vi "StartData.vi"(8 "error in (no error)":errorcluster, 11 "Class In":refnum<class "C37.118 PMU.lvclass">) -> (0 "error out":errorcluster, 3 "Class Out":refnum<class "C37.118 PMU.lvclass">)   [LabVIEW 2014, in "SensorPlugins.lvlib" / "C37.118 PMU.lvclass"]
uses:
  C37.118 PMU.lvclass
  Typedef/eCmdTypes.ctl
  C37.118 PMU.lvclass/C37.118 PMU.ctl
  <userlib>/NIST/Socket Class/Classes/Socket.Base/Socket.Base.lvclass/Socket.Base.ctl
  <userlib>/NIST/Socket Class/Classes/Socket.Base/Accessors/Read connected.vi
  Accessors/Read PMUConfigData.vi
  Accessors/Read CmdSocket.vi
  Accessors/Read PMUComms.vi
  Accessors/Read DataSocket.vi
  Accessors/Write CmdSocket.vi
  Accessors/Write DataSocket.vi
  <userlib>/NIST/Socket Class/Classes/Socket.Base/Socket.Base.lvclass
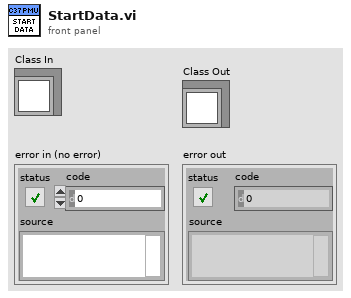
[diagram p1: front panel]
types:
  T1 = typedef "SensorPlugins.lvlib/C37.118 PMU.lvclass/eCmdTypes.ctl" = enum16{"Stop realtime data", "Start realtime data", "Send HDR file", "Send CFG-1 file", "Send CFG-2 file"}
  T2 = typedef "SensorPlugins.lvlib/C37.118 PMU.lvclass/PMUConfigData.ctl" = cluster{"TimeBase":u32, "NUM_PMU":u16, "Station Name":string, "IDCODE":u16, "PHRNMR":u16, "ANNMR":u16, "DIGNMR":u16, "FORMAT BITS":T3, "Valid Inputs":u16[], "DigitalStatusMask":u16[], "24bit_PHUNIT":i32[], "24bit_ANUNIT":u32[], "Analog Amplitude Setting":u32[], "Unit (Vor I)":u8[], "ChannelNames":string, "Fs":i16, "SOC ":u32, "FRACSEC":u32, "F0":sgl, "CFGCNT":u16}
  T3 = typedef "SensorPlugins.lvlib/C37.118 PMU.lvclass/FormatBits.ctl" = cluster{"Rect/Polar":bool, "Phasor Int/Float":bool, "Analog Int/Float":bool, "F/ROCOF Int/Float":bool}
  T4 = typedef "SensorPlugins.lvlib/C37.118 PMU.lvclass/PMUComms.ctl" = cluster{"PMU IP Address":string, "CMD Comms Type":T5, "Data Comms Type":T5, "CMD Port":u16, "Data Port":u16, "PMU ID":u16}
  T5 = typedef "SensorPlugins.lvlib/C37.118 PMU.lvclass/eCommsType.ctl" = enum16{"TCP", "UDP", "USB", "GPIB"}
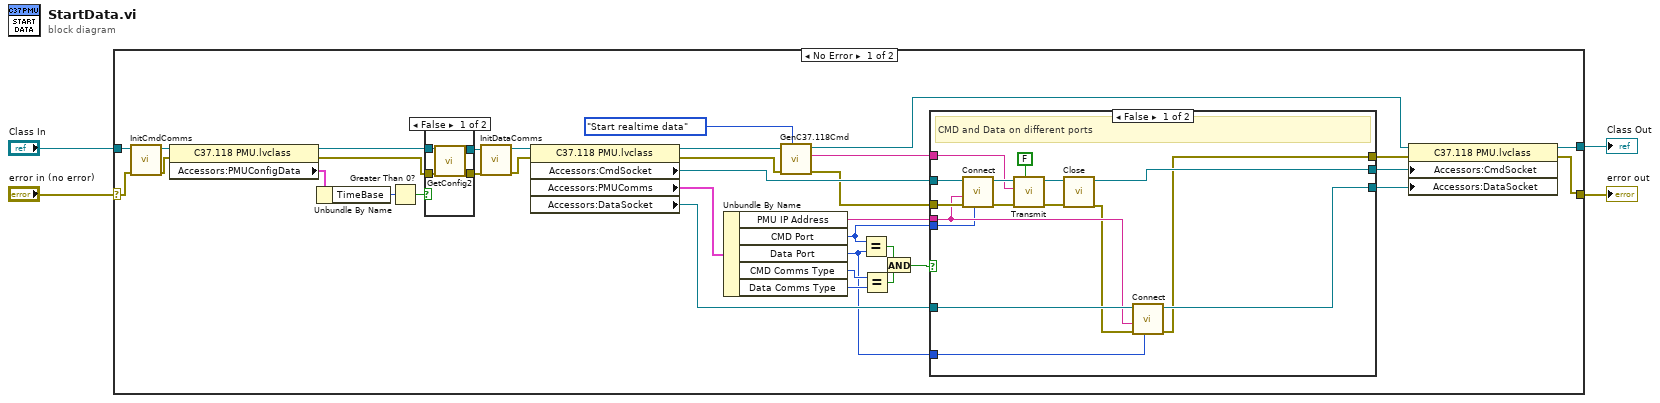
[diagram p0: block diagram]
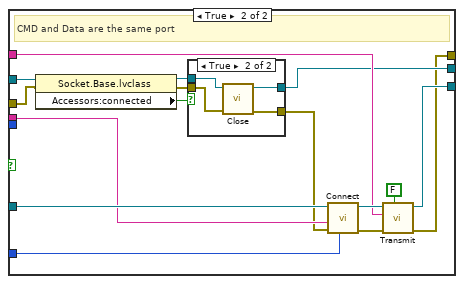
[diagram p3: hidden frame]
diagram:
  n1 = case shown="No Error" "error in (no error)" {
    selector: "error in (no error)" -> [w32 w84]
    tunnel: "Class In" -> [w33 w85]
    tunnel: [w28 w85] -> w2
    tunnel: [w23 w84] -> w1
    frame No Error {
      n2 = call "InitCmdComms.vi"("error in (no error)"=w32, "C37.118 PMU in"=w33) -> ("error out"=w7:errorcluster, "C37.118 PMU out"=w31:refnum<class "C37.118 PMU.lvclass">)  [unwired: 8 in]
      n3 = property class="C37.118 PMU.lvclass"(reference=w31, error in=w7) -> (reference out=w10:refnum<class "C37.118 PMU.lvclass">, error out=w6:errorcluster, "Accessors:PMUConfigData"=w12:T2)
      n4 = Unbundle By Name(w12) -> ("TimeBase"=w9:u32)
      n5 = Greater Than 0?(x=w9) -> (x > 0?=w8:bool)
      n6 = case shown="False" w8 {
        tunnel: [w43 w45] -> w11
        tunnel: w10 -> [w42 w45]
        tunnel: w6 -> [w41 w44]
        tunnel: [w40 w44] -> w5
        frame False {
          n7 = call "GetConfig2.vi"("error in (no error)"=w41, "C37.118 PMU in"=w42) -> ("error out"=w40:errorcluster, "C37.118 PMU out"=w43:refnum<class "C37.118 PMU.lvclass">)  [unwired: 8 in]
        }
        frame True {
        }
      }
      n8 = call "InitDataComms.vi"("error in (no error)"=w5, "C37.118 PMU in"=w11) -> ("error out"=w29:errorcluster, "C37.118 PMU out"=w30:refnum<class "C37.118 PMU.lvclass">)  [unwired: 8 in]
      n9 = property class="C37.118 PMU.lvclass"(reference=w30, error in=w29) -> (reference out=w38:refnum<class "C37.118 PMU.lvclass">, error out=w25:errorcluster, "Accessors:CmdSocket"=w37:refnum<class "Socket.Base.lvclass">, "Accessors:PMUComms"=w36:T4, "Accessors:DataSocket"=w26:refnum<class "Socket.Base.lvclass">)
      n10 = Unbundle By Name(w36) -> ("PMU IP Address"=w24:string, "CMD Port"=w15:u16, "Data Port"=w14:u16, "CMD Comms Type"=w20:T5, "Data Comms Type"=w19:T5)
      n11 = call "GenC37.118Cmd.vi"("Function"=eCmdTypes."Start realtime data", "error in (no error)"=w25, "PMUClass"=w38) -> ("error out"=w34:errorcluster, "Command"=w35:string, "PMUClass"=w13:refnum<class "C37.118 PMU.lvclass">)  [unwired: 6 in]
      n12 = Equal?(x=w15, y=w14) -> (x = y?=w18:bool)
      n13 = Equal?(x=w20, y=w19) -> (x = y?=w17:bool)
      n14 = And(x=w18, y=w17) -> (x .and. y?=w16:bool)
      n15 = case shown="False" w16 {
        tunnel: w37 -> [w61 w71]
        tunnel: w35 -> [w57 w72]
        tunnel: w34 -> [w56 w70]
        tunnel: [w53 w66] -> w27
        tunnel: w26 -> [w52 w77]
        tunnel: w24 -> [w51 w75]
        tunnel: [w50 w63] -> w22
        tunnel: [w48 w62] -> w21
        tunnel: w15 -> [w47 _]
        tunnel: w14 -> [w46 w76]
        frame False {
          # "CMD and Data on different ports"
          n16 = call-dynamic "Connect.vi"("remote_port"=w47, "error in (no error)"=w56, "remote_address"=w51, "Socket.Base in"=w61) -> ("error out"=w58:errorcluster, "Socket.Base out"=w59:refnum<class "Socket.Base.lvclass">)  [unwired: 6 in]
          n17 = call-dynamic "Transmit.vi"("packet? (f)"=FALSE, "error in (no error)"=w58, "data"=w57, "Socket.Base in"=w59) -> ("error out"=w55:errorcluster, "Socket.Base out"=w54:refnum<class "Socket.Base.lvclass">)  [unwired: 5 in, 1 out]
          n18 = call-dynamic "Close.vi"("error in (no error)"=w55, "Socket.Base in"=w54) -> ("error out"=w49:errorcluster, "Socket.Base out"=w53:refnum<class "Socket.Base.lvclass">)  [unwired: 8 in]
          n19 = call-dynamic "Connect.vi"("remote_port"=w46, "error in (no error)"=w49, "remote_address"=w51, "Socket.Base in"=w52) -> ("error out"=w48:errorcluster, "Socket.Base out"=w50:refnum<class "Socket.Base.lvclass">)  [unwired: 6 in]
        }
        frame True {
          # "CMD and Data are the same port"
          n20 = property class="Socket.Base.lvclass"(reference=w71, error in=w70) -> (reference out=w68:refnum<class "Socket.Base.lvclass">, error out=w67:errorcluster, "Accessors:connected"=w69:bool)
          n21 = case shown="True" w69 {
            tunnel: w68 -> [w79 w83]
            tunnel: w67 -> [w78 w82]
            tunnel: [w78 w81] -> w65
            tunnel: [w79 w80] -> w66
            frame False {
            }
            frame True {
              n22 = call-dynamic "Close.vi"("error in (no error)"=w82, "Socket.Base in"=w83) -> ("error out"=w81:errorcluster, "Socket.Base out"=w80:refnum<class "Socket.Base.lvclass">)  [unwired: 8 in]
            }
          }
          n23 = call-dynamic "Connect.vi"("remote_port"=w76, "error in (no error)"=w65, "remote_address"=w75, "Socket.Base in"=w77) -> ("error out"=w74:errorcluster, "Socket.Base out"=w73:refnum<class "Socket.Base.lvclass">)  [unwired: 6 in]
          n24 = call-dynamic "Transmit.vi"("packet? (f)"=FALSE, "error in (no error)"=w74, "data"=w72, "Socket.Base in"=w73) -> ("error out"=w62:errorcluster, "Socket.Base out"=w63:refnum<class "Socket.Base.lvclass">)  [unwired: 5 in, 1 out]
        }
      }
      n25 = property class="C37.118 PMU.lvclass"(reference=w13, error in=w21, "Accessors:CmdSocket"=w27, "Accessors:DataSocket"=w22) -> (reference out=w28:refnum<class "C37.118 PMU.lvclass">, error out=w23:errorcluster)
    }
    frame Error {
    }
  }
  "Class Out" <- w2
  "error out" <- w1
